vi "Read Lock State.vi"(8 "error in (no error)":errorcluster, 11 "protection settings in":refnum<class "protection settings.lvclass">) -> (0 "error out":errorcluster, 2 "Lock State":T1(ring)=enum."Locked (No Password)", 3 "protection settings out":refnum<class "protection settings.lvclass">)   [LabVIEW 2013, in "protection settings.lvclass"]
uses:
  protection settings.lvclass
  protection settings.lvclass/protection settings.ctl
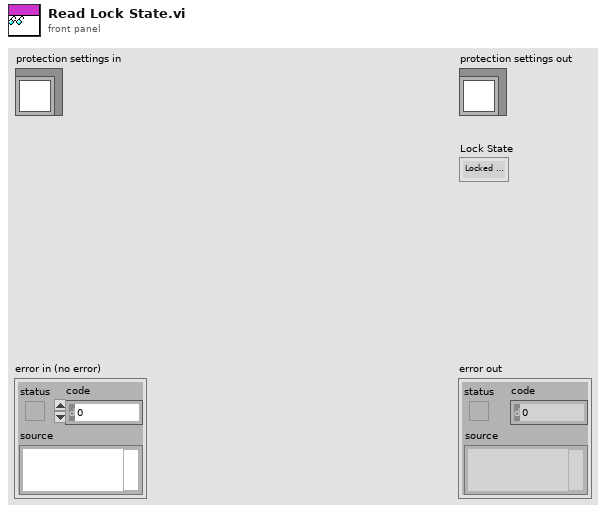
[diagram p1: front panel]
types:
  T1 = enum32{"invalid lock state", "Not Locked", "Locked (No Password)", "Password-protected"}
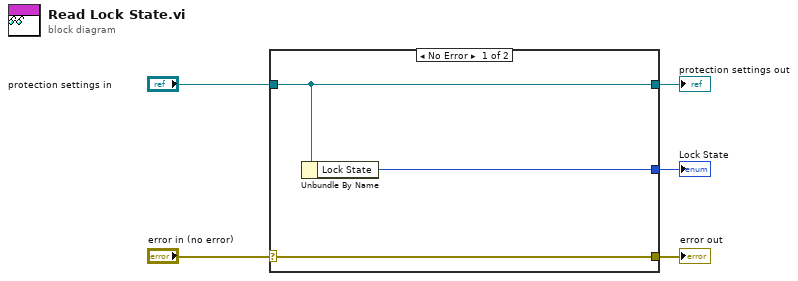
[diagram p0: block diagram]
diagram:
  n1 = case shown="No Error" "error in (no error)" {
    selector: "error in (no error)" -> [w8 w9]
    tunnel: [w8 w9] -> w4
    tunnel: [w7 w10] -> w2
    tunnel: "protection settings in" -> [w7 w10]
    tunnel: [w6 _] -> w1
    frame No Error {
      n2 = Unbundle By Name(w7) -> ("Lock State"=w6:T1)
    }
    frame Error {
    }
  }
  "error out" <- w4
  "protection settings out" <- w2
  "Lock State" <- w1
